vi "Initialize.vi"(8 "error in":errorcluster, 11 "VISA resource name":refnum<visa-resource-name>="COM1") -> (0 "error out":errorcluster, 3 "reference out":refnum<visa-resource-name>)   [LabVIEW 2011]
uses:
  <vilib>/Instr/_visa.llb/VISA Configure Serial Port (Instr).vi
panel:
  in  "timeout (ms)":u32=10000
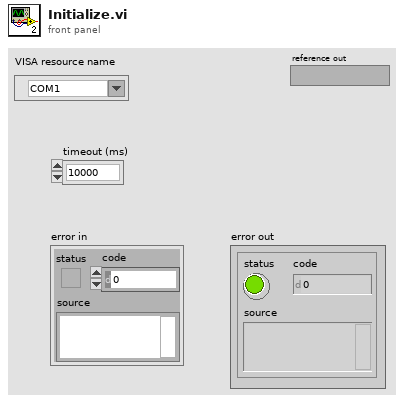
[diagram p1: front panel]
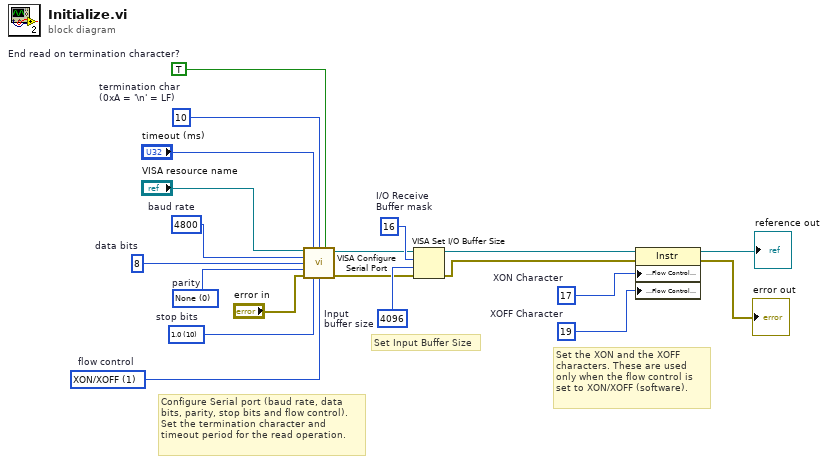
[diagram p0: block diagram]
diagram:
  w15 = TRUE  # End read on termination character?
  w7 = u8 19  # XOFF Character
  w8 = u8 17  # XON Character
  w13 = u32 4096  # Input buffer size
  w11 = u16 1 items=["None"=0, "XON/XOFF"=1, "RTS/CTS"=2, "DTR/DSR"=4]  # flow control
  w17 = u16 10 items=["1.0"=10, "1.5"=15, "2.0"=20]  # stop bits
  w18 = u16 0 items=["None", "Odd", "Even", "Mark", "Space"]  # parity
  w6 = u16 8  # data bits
  w20 = u32 4800  # baud rate
  w12 = u8 10  # termination char (0xA = '\n' = LF)
  w14 = u16 16  # I/O Receive Buffer mask
  # "Set the XON and the XOFF\ncharacters. These are used\nonly when the flow control is\nset to XON/XOFF (software)."
  # "Configure Serial port (baud rate, data\nbits, parity, stop bits and flow control).\nSet the termination character and\ntimeout period for the read operation."
  # "Set Input Buffer Size"
  n1 = call-poly "VISA Configure Serial Port"("VISA resource name"="VISA resource name", "timeout (10sec)"="timeout (ms)", "termination char\n(0xA = '\\n' = LF)"=w12, "Enable Termination\nChar (T)"=w15, "baud rate (9600)"=w20, "data bits (8)"=w6, "parity (0:none)"=w18, "error in (no error)"="error in", "stop bits (10: 1 bit)"=w17, "flow control (0:none)"=w11) -> ("VISA resource name out"=w4:refnum<visa-resource-name>, "error out"=w3:errorcluster)  [unwired: 4 in]
  n2 = VISA Set I/O Buffer Size(VISA resource name=w4, mask (16)=w14, size (4096)=w13, error in (no error)=w3) -> (VISA resource name out=w10:refnum<visa-resource-name>, error out=w9:errorcluster)
  n3 = property class="Instr"(reference=w10, error in=w9, "Serial Settings:Flow Control XON Character"=w8, "Serial Settings:Flow Control XOFF Character"=w7) -> (reference out=→"reference out":refnum<visa-resource-name>, error out=→"error out":errorcluster)
